vi "PH_Sixpack.Set Position.vi"(0 "i ref in":refnum<vi>, 1 "axis":i32=-1, 2 "Position to set":i32, 4 "Device Error in":errorcluster, 5 "error in":errorcluster) -> (14 "i ref out":refnum<vi>, 16 "ok?":bool, 18 "Device Error out":errorcluster, 19 "error out":errorcluster)   [LabVIEW 2014, in "PH_Sixpack.lvlib"]
doc: "This VI acts on the hardware."
uses:
  PH_Sixpack.lvlib
  instr.lib/Sixpack/Sixpack - Driver.lvlib
  PH_Basics/PH_Stepmotor_BaseClass/PH_Stepmotor_BaseClass.lvlib
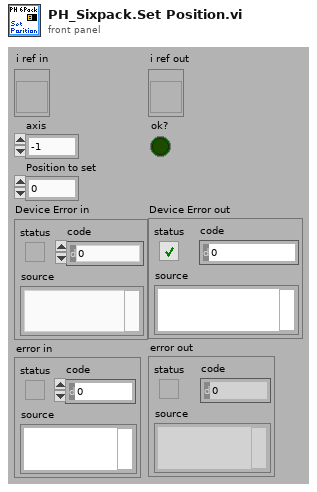
[diagram p1: front panel]
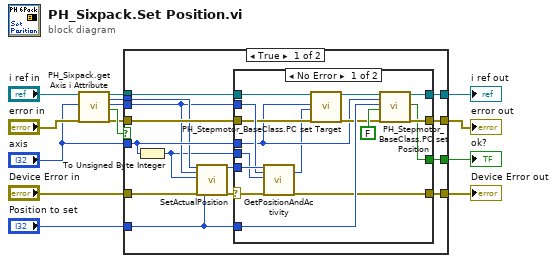
[diagram p0: block diagram]
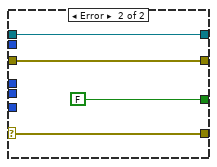
[diagram p2: hidden frame]
diagram:
  n1 = call "PH_Sixpack.get Axis i Attribute.vi"("VI in"="i ref in", "Axis"="axis", "error in"="error in") -> ("VI out"=w9:refnum<vi>, "HANDLE"=w6:i32, "SixPack ID(0)"=w5:u16, "Axis found?"=w12:bool, "error out"=w11:errorcluster)  [unwired: 10 in, 2 out]
  n2 = case shown="True" w12 {
    tunnel: [w25 w52] -> w10
    tunnel: w11 -> [w28 w52]
    tunnel: [w26 w51] -> w8
    tunnel: w9 -> [w27 w51]
    tunnel: "Position to set" -> [w22 _]
    tunnel: "axis" -> [w23 _]
    tunnel: w6 -> [w18 _]
    tunnel: w5 -> [w16 _]
    tunnel: [w19 w50] -> w4
    tunnel: "Device Error in" -> [w24 w50]
    tunnel: [w20 TRUE] -> w1
    frame True {
      n3 = To Unsigned Byte Integer(number=w23) -> (unsigned 8bit integer=w15:u8)
      n4 = call "SetActualPosition.vi"("handle in"=w18, "UnitAddress(0)"=w16, "MotNr(0)"=w15, "error in"=w24, "ActualPosition(0)"=w22) -> ("handle out"=w17:i32, "error out"=w21:errorcluster)  [unwired: 13 in]
      n5 = case shown="No Error" w21 {
        selector: w21 -> [w39 w45]
        tunnel: w28 -> [w34 w47]
        tunnel: w27 -> [w32 w48]
        tunnel: [w44 w48] -> w26
        tunnel: [w43 w47] -> w25
        tunnel: w23 -> [w30 _]
        tunnel: w22 -> [w41 _]
        tunnel: [w40 FALSE] -> w20
        tunnel: [w38 w45] -> w19
        tunnel: w17 -> [w37 _]
        tunnel: w16 -> [w36 _]
        tunnel: w15 -> [w35 _]
        frame No Error {
          n6 = call "GetPositionAndActivity.vi"("handle in"=w37, "UnitAddress(0)"=w36, "MotNr(0)"=w35, "error in"=w39) -> ("CurrentPosition"=w29:i32, "error out"=w38:errorcluster)  [unwired: 11 in, 3 out]
          n7 = call "PH_Stepmotor_BaseClass.PC set Target.vi"("VI in"=w32, "axis"=w30, "Targetposition to set"=w29, "error in (no error)"=w34) -> ("VI out"=w31:refnum<vi>, "error out"=w33:errorcluster)  [unwired: 14 in]
          n8 = call "PH_Stepmotor_BaseClass.PC set Position.vi"("i ref in"=w31, "axis"=w30, "Position to set"=w41, "Set?"=FALSE, "error in (no error)"=w33) -> ("i ref out"=w44:refnum<vi>, "ok?"=w40:bool, "error out"=w43:errorcluster)  [unwired: 12 in]
        }
        frame Error {
        }
      }
    }
    frame False {
    }
  }
  "error out" <- w10
  "i ref out" <- w8
  "Device Error out" <- w4
  "ok?" <- w1
